vi "code_loop.vi"(0 "heat_board_control in":refnum<class "heat_board_control.lvclass">, 1 "laser setpoint in":dbl, 4 "millisecond\n multiple":u32, 5 "lock all":bool, 7 "error in (no error)":errorcluster, 11 "sampling info":cluster{"Fs":dbl, "#s":dbl}={"Fs"=5000.0, "#s"=1000.0} {"Fs" format="%.2p"}) -> (20 "heat_board_control out":refnum<class "heat_board_control.lvclass">, 23 "data average":dbl, 24 "PD setpoint":dbl, 25 "laser setpoint out":dbl, 26 "Boolean":bool, 27 "error out":errorcluster)   [LabVIEW 2015, in "heat_board_control.lvclass"]
uses:
  heat_board_control.lvclass
  <vilib>/DAQmx/read.llb/DAQmx Read (Analog Wfm 1Chan NSamp).vi
  <vilib>/ULx/Write.llb/ULx Write (Analog 1D DBL 1Chan 1Samp).vi
  <vilib>/DAQmx/miscellaneous.llb/DAQmx Fill In Error Info.vi
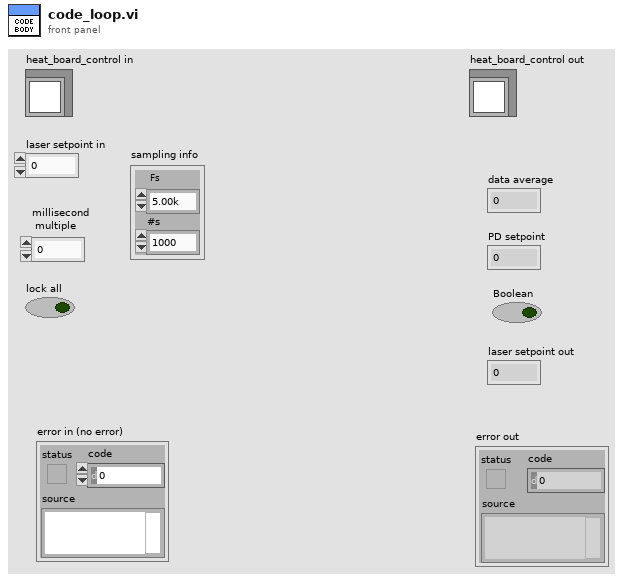
[diagram p1: front panel]
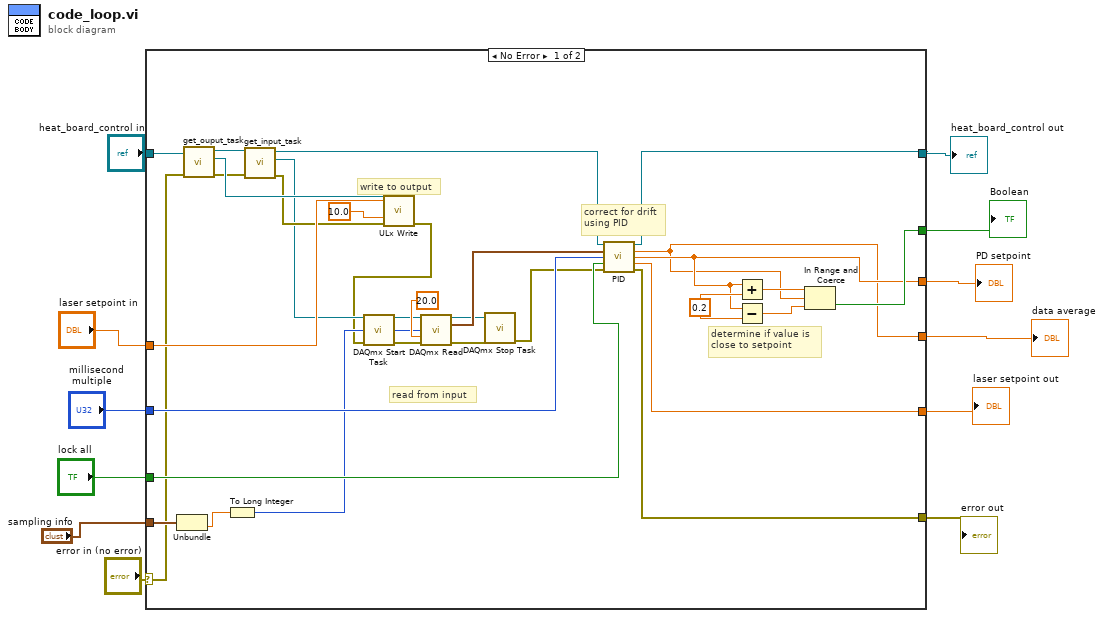
[diagram p0: block diagram]
diagram:
  n1 = case shown="No Error" "error in (no error)" {
    selector: "error in (no error)" -> [w22 w46]
    tunnel: [w36 w46] -> w11
    tunnel: [w40 w45] -> w9
    tunnel: "heat_board_control in" -> [w26 w45]
    tunnel: "laser setpoint in" -> [w39 _]
    tunnel: "millisecond\n multiple" -> [w38 _]
    tunnel: "lock all" -> [w37 _]
    tunnel: [w35 _] -> w5
    tunnel: [w34 _] -> w4
    tunnel: [w33 _] -> w3
    tunnel: [w32 _] -> w2
    tunnel: "sampling info" -> [w28 _]
    frame No Error {
      w43 = 0.2
      # "determine if value is \nclose to setpoint"
      # "correct for drift\nusing PID"
      # "read from input"
      # "write to output"
      n2 = Unbundle(w28) -> ("#s"=w29:dbl)  [unwired: 1 out]
      n3 = call-dynamic "get_ouput_task.vi"("error in (no error)"=w22, "heat_board_control in"=w26) -> ("error out"=w23:errorcluster, "output task out"=w25:refnum<k24>, "heat_board_control out"=w24:refnum<class "heat_board_control.lvclass">)  [unwired: 7 in]
      n4 = To Long Integer(number=w29) -> (32bit integer=w27:i32)
      n5 = call-dynamic "get_input_task.vi"("error in (no error)"=w23, "heat_board_control in"=w24) -> ("error out"=w21:errorcluster, "input task out"=w19:refnum<k21>, "heat_board_control out"=w20:refnum<class "heat_board_control.lvclass">)  [unwired: 7 in]
      n6 = call-poly <vilib>:"ULx Write.vi"("task in"=w25, "data"=w39, "timeout"=10.0, "error in"=w21) -> ("error out"=w17:errorcluster)  [unwired: 9 in, 2 out]
      n7 = call <vilib>:"DAQmx Start Task.vi"("task/channels in"=w19, "error in"=w17) -> ("task out"=w18:refnum<k21>, "error out"=w16:errorcluster)  [unwired: 12 in]
      n8 = call-poly <vilib>:"DAQmx Read.vi"("task/channels in"=w18, "number of samples per channel"=w27, "timeout"=20.0, "error in"=w16) -> ("task out"=w15:refnum<k21>, "data"=w30:waveform(dbl), "error out"=w14:errorcluster)  [unwired: 9 in]
      n9 = call <vilib>:"DAQmx Stop Task.vi"("task/channels in"=w15, "error in"=w14) -> ("error out"=w13:errorcluster)  [unwired: 12 in, 1 out]
      n10 = call-dynamic "PID.vi"("heat_board_control in"=w20, "Waveform"=w30, "millisecond multiple"=w38, "Lock All"=w37, "error in (no error)"=w13) -> ("heat_board_control out"=w40:refnum<class "heat_board_control.lvclass">, "data average"=w32:dbl, "PD setpoint"=w33:dbl, "laser setpoint"=w35:dbl, "error out"=w36:errorcluster)  [unwired: 6 in]
      n11 = Add(x=w33, y=w43) -> (x+y=w42:dbl)
      n12 = Subtract(x=w33, y=w43) -> (x-y=w41:dbl)
      n13 = In Range and Coerce(upper limit=w42, x=w32, lower limit=w41) -> (In Range?=w34:bool)  [unwired: 1 out]
    }
    frame Error {
    }
  }
  "error out" <- w11
  "heat_board_control out" <- w9
  "laser setpoint out" <- w5
  "Boolean" <- w4
  "PD setpoint" <- w3
  "data average" <- w2
